vi "Write Number of Sensors.vi"(8 "error in (no error)":errorcluster, 10 "Number of Sensors":u16[](array[numeric]), 11 "Micron Optics Driver in":refnum<class "Micron Optics Driver.lvclass">) -> (0 "error out":errorcluster, 3 "Micron Optics Driver out":refnum<class "Micron Optics Driver.lvclass">)   [LabVIEW 2024, in "Micron Optics Driver.lvclass"]
uses:
  Micron Optics Driver.lvclass
  Micron Optics Driver.lvclass/Micron Optics Driver.ctl
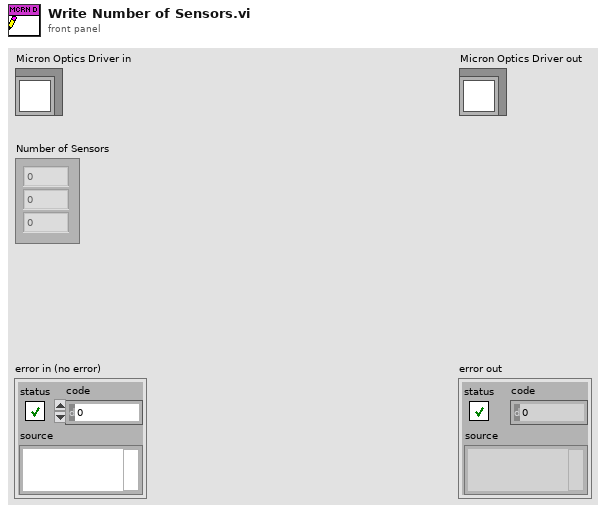
[diagram p1: front panel]
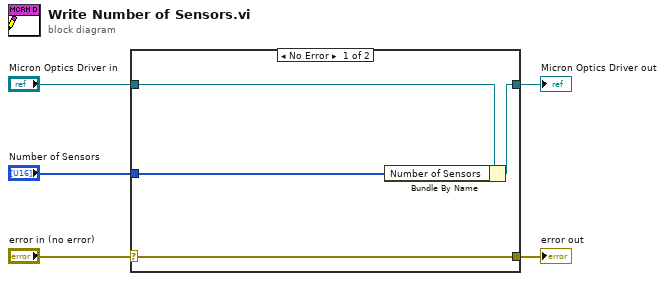
[diagram p0: block diagram]
diagram:
  n1 = case shown="No Error" "error in (no error)" {
    selector: "error in (no error)" -> [w9 w10]
    tunnel: [w9 w10] -> w4
    tunnel: [w7 w11] -> w2
    tunnel: "Micron Optics Driver in" -> [w8 w11]
    tunnel: "Number of Sensors" -> [w6 _]
    frame No Error {
      n2 = Bundle By Name(cluster=w8, "Number of Sensors"=w6) -> (w7:refnum<class "Micron Optics Driver.lvclass">)
    }
    frame Error {
    }
  }
  "error out" <- w4
  "Micron Optics Driver out" <- w2
